vi "Counter.vi"() -> ()   [LabVIEW 2016]
panel:
  out "波形图表":dbl(graph)
  out "error out":errorcluster caption="错误输出"
  out "CtrN":u32[](array[numeric])
  out "CtrT(us)":dbl[](array[numeric]) format="%#.6g"
  in  "停止":bool
  in  "CtrEdge":u8(ring)=1 items=["上升沿"=1, "下降沿"=2]
  in  "CtrMode":u8(ring) items=["计数器", "周期", "正脉宽", "负脉宽"]
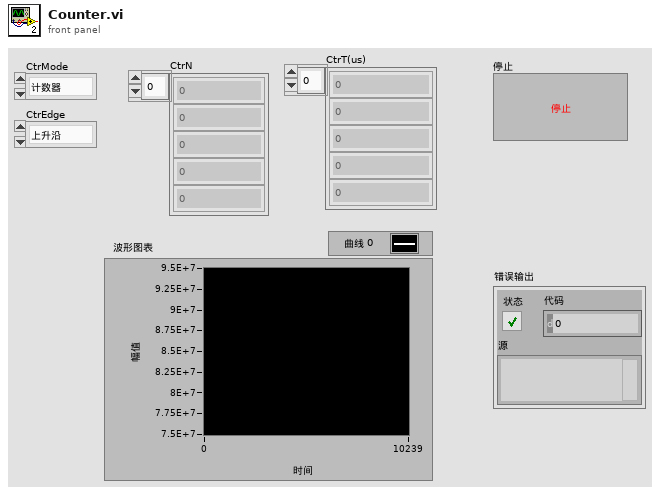
[diagram p1: front panel]
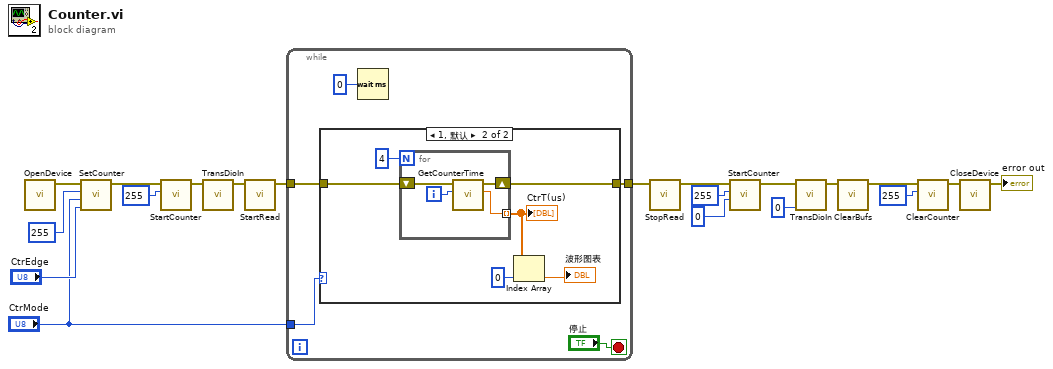
[diagram p0: block diagram]
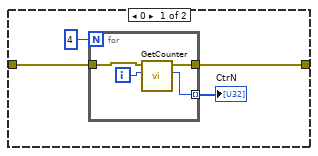
[diagram p2: hidden frame]
diagram:
  n1 = call "OpenDevice.vi"() -> ("error out"=w20:errorcluster)  [unwired: 11 in]
  n2 = call "SetCounter.vi"("CtrEdge"="CtrEdge", "CtrMode"="CtrMode", "CtrNum"=u8 255, "error in"=w20) -> ("error out"=w13:errorcluster)  [unwired: 7 in]
  n3 = call "StartCounter.vi"("CtrNum"=u8 255, "error in"=w13) -> ("error out"=w12:errorcluster)  [unwired: 9 in]
  n4 = call "TransDioIn.vi"("error in"=w12) -> ("error out"=w19:errorcluster)  [unwired: 10 in]
  n5 = call "StartRead.vi"("error in"=w19) -> ("error out"=w18:errorcluster)  [unwired: 10 in]
  n6 = while {
    tunnel: w18 -> [w24]
    tunnel: "CtrMode" -> [w25]
    tunnel: [w23] -> w15
    stop <- "停止" stop-if-true
    n7 = case shown="1, 默认" w25 {
      tunnel: w24 -> [w29 w39]
      tunnel: [w28 w38] -> w23
      frame 0 {
        n8 = for {
          N: 4 -> [_]
          tunnel: [w30] -> w26 mode=indexing
          tunnel: w29 -> [w33]
          tunnel: [w32] -> w28
          i -> [w31]
          n9 = call "GetCounter.vi"("CtrNum"=w31, "error in"=w33) -> ("Counter"=w30:u32, "error out"=w32:errorcluster)  [unwired: 8 in]
        }
        "CtrN" <- w26
      }
      frame 1, Default {
        n10 = for {
          N: 4 -> [_]
          shift-right: [w42] -> w38
          shift-left: w39 -> [w43]
          tunnel: [w40] -> w36 mode=indexing
          i -> [w41]
          n11 = call "GetCounterTime.vi"("CtrNum"=w41, "error in"=w43) -> ("CounterTime"=w40:dbl, "error out"=w42:errorcluster)  [unwired: 8 in]
        }
        "CtrT(us)" <- w36
        n12 = Index Array(array=w36, index=0 ("索引")) -> (element=→"波形图表":dbl)
      }
    }
    n13 = Wait (ms)(milliseconds to wait=u32 0 ("等待时间（毫秒）")) -> ()  [unwired: 1 out]
  }
  n14 = call "StopRead.vi"("error in"=w15) -> ("error out"=w3:errorcluster)  [unwired: 10 in]
  n15 = call "StartCounter.vi"("OnOff"=u8 0, "CtrNum"=u8 255, "error in"=w3) -> ("error out"=w2:errorcluster)  [unwired: 8 in]
  n16 = call "TransDioIn.vi"("TransDioInSwitch"=u8 0, "error in"=w2) -> ("error out"=w5:errorcluster)  [unwired: 9 in]
  n17 = call "ClearBufs.vi"("error in"=w5) -> ("error out"=w1:errorcluster)  [unwired: 10 in]
  n18 = call "ClearCounter.vi"("CtrNum"=u8 255, "error in"=w1) -> ("error out"=w4:errorcluster)  [unwired: 9 in]
  n19 = call "CloseDevice.vi"("error in"=w4) -> ("error out"=→"error out":errorcluster)  [unwired: 10 in]
